vi "3446X_Initialize.vi"(0 "Instrument Info":T1, 1 "User Reference":i32, 5 "error in (no error)":errorcluster) -> (19 "error out":errorcluster)   [LabVIEW 2018, in "3446X.lvclass"]
uses:
  3446X.lvclass
  Station/Station Support/Controls/Instrument Info.ctl
  C:/Users/John Gmitter/OneDrive - National Instruments/Git Repo/Harris-FL/Reference Management Server/Instrument Drivers/DMM/DMM Virtual/DMM Virtual.lvclass
  3446X.lvclass/3446X.ctl
  DMM Virtual/DMM Virtual.lvclass
  <instrlib>/Agilent 3446X Series/Agilent 3446X Series.lvlib
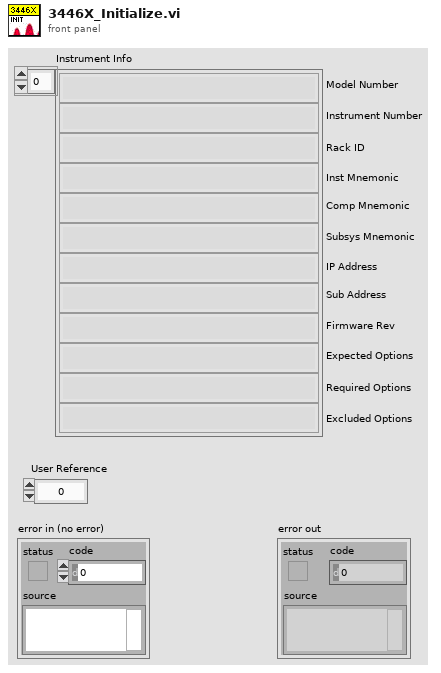
[diagram p1: front panel]
types:
  T1 = typedef "Instrument Info.ctl" = string[]
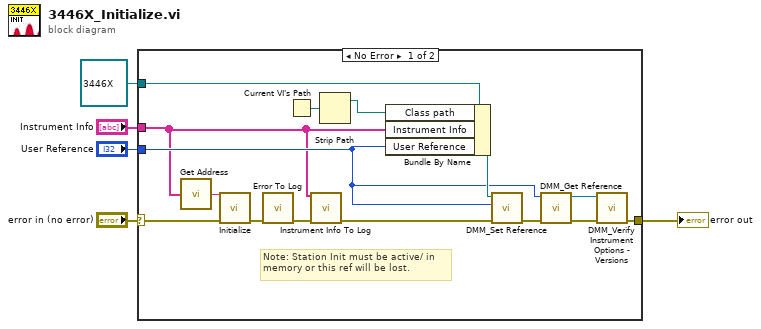
[diagram p0: block diagram]
diagram:
  n1 = case shown="No Error" "error in (no error)" {
    selector: "error in (no error)" -> [w10 w21]
    tunnel: [w16 w21] -> w2
    tunnel: refnum<class "3446X.lvclass"> refnum ("3446X in") -> [w20 _]
    tunnel: "Instrument Info" -> [w8 _]
    tunnel: "User Reference" -> [w14 _]
    frame No Error {
      # "Note: Station Init must be active/ in\nmemory or this ref will be lost."
      n2 = call "Get Address.vi"("Instrument Info"=w8) -> ("Address"=w9:string)  [unwired: 4 in]
      n3 = call <instrlib>:"Initialize.vi"("error in (no error)"=w10, "VISA resource name"=w9) -> ("error out"=w11:errorcluster)  [unwired: 8 in, 1 out]
      n4 = call "Error To Log.vi"("error in (no error)"=w11) -> ("error out"=w13:errorcluster)  [unwired: 14 in]
      n5 = Current VI's Path() -> (path=w7:path)
      n6 = call "Instrument Info To Log.vi"("Instrument Info"=w8, "error in (no error)"=w13) -> ("error out"=w12:errorcluster)  [unwired: 13 in]
      n7 = Strip Path(path=w7) -> (stripped path=w6:path)  [unwired: 1 out]
      n8 = Bundle By Name(cluster=w20, "Class path"=w6, "Instrument Info"=w8, "User Reference"=w14) -> (w19:refnum<class "3446X.lvclass">)
      n9 = call "DMM_Set Reference.vi"("error in (no error)"=w12, "Instrument Reference"=w14, "DMM Virtual in"=w19) -> ("error out"=w18:errorcluster)  [unwired: 8 in]
      n10 = call "DMM_Get Reference.vi"("error in (no error)"=w18, "Instrument Reference"=w14) -> ("error out"=w17:errorcluster, "DMM Virtual.lvclass"=w15:refnum<class "DMM Virtual.lvclass">)  [unwired: 7 in, 1 out]
      n11 = call-dynamic "DMM_Verify Instrument Options - Versions.vi"("error in (no error)"=w17, "DMM Virtual in"=w15) -> ("error out"=w16:errorcluster)  [unwired: 8 in, 1 out]
    }
    frame Error {
    }
  }
  "error out" <- w2
